vi "TEMPERATUTA.vi"(10 "TK/TC":bool, 11 "Tf":dbl) -> (3 "TC":dbl)   [LabVIEW 2018]
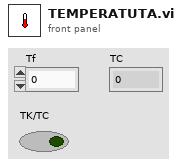
[diagram p1: front panel]
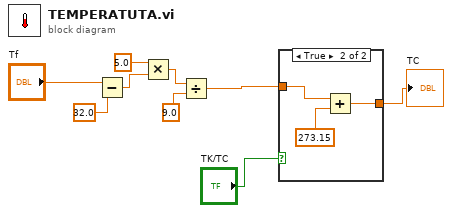
[diagram p0: block diagram]
diagram:
  n1 = Subtract(x="Tf", y=32.0 ("x-y")) -> (x-y=w3:dbl)
  n2 = Multiply(x=5.0, y=w3) -> (x*y=w5:dbl)
  n3 = Divide(x=w5, y=9.0 ("x-y")) -> (x/y=w7:dbl)
  n4 = case shown="True" "TK/TC" {
    tunnel: w7 -> [w10 w13]
    tunnel: [w10 w11] -> w8
    frame False {
    }
    frame True {
      n5 = Add(x=w13, y=273.15 ("x+y")) -> (x+y=w11:dbl)
    }
  }
  "TC" <- w8
